vi "Set Legend (XYGraph).vi"(8 "error in (no error)":errorcluster, 9 "Plot.Plot Name":string, 10 "Active Plot":i32, 11 "XYGraph in":refnum<vi>) -> (0 "error out":errorcluster, 1 "Plot.Plot Name":string, 2 "Active Plot":i32, 3 "XYGraph out":refnum<vi>)   [LabVIEW 2019, in "Instrument UI.Lockin.lvclass"]
uses:
  Instrument UI.Lockin.lvclass
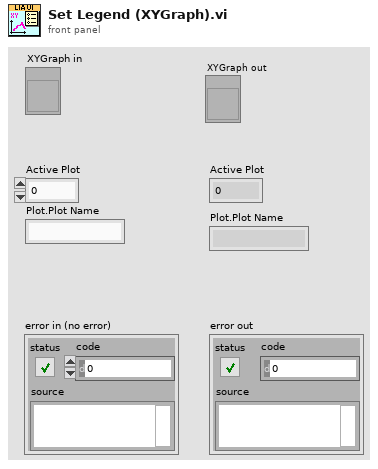
[diagram p1: front panel]
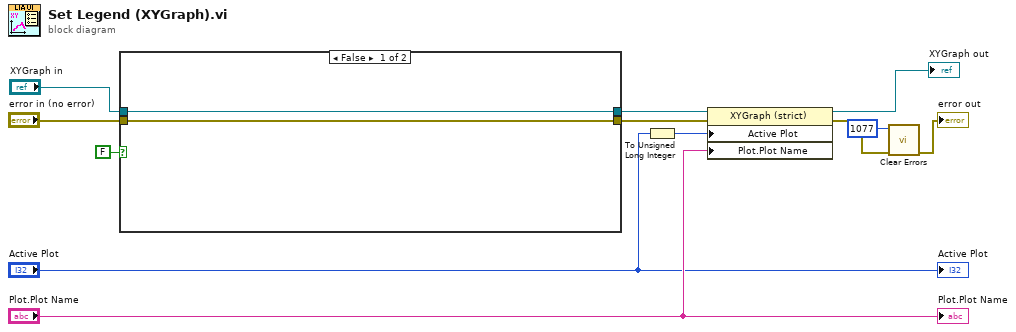
[diagram p0: block diagram]
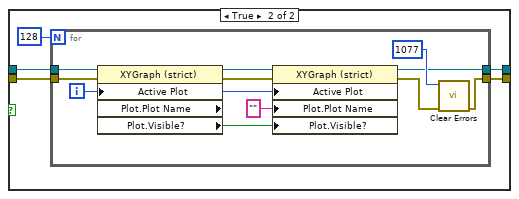
[diagram p2: hidden frame]
diagram:
  n1 = case shown="False" FALSE {
    tunnel: "XYGraph in" -> [w13 w16]
    tunnel: [w14 w19] -> w4
    tunnel: "error in (no error)" -> [w14 w18]
    tunnel: [w13 w15] -> w5
    frame False {
    }
    frame True {
      n2 = for {
        N: 128 -> [_]
        tunnel: w16 -> [w23]
        tunnel: [w28] -> w19
        tunnel: w18 -> [w22]
        tunnel: [w26] -> w15
        i -> [w21]
        n3 = property on="Property Node" class="XYGraph (strict)" props=["Active Plot", "Plot", "Plot Name", "Plot", "Visible?"](reference=w23, error in=w22, "Active Plot"=w21) -> (reference out=w25:refnum<vi>, error out=w24:errorcluster, "Plot.Visible?"=w20:bool)  [unwired: 1 out]
        n4 = property on="Property Node" class="XYGraph (strict)"(reference=w25, error in=w24, "Active Plot"=w21, "Plot.Plot Name"="" ("format string"), "Plot.Visible?"=w20) -> (reference out=w26:refnum<vi>, error out=w29:errorcluster)
        n5 = call <vilib>:"Clear Errors.vi"("error in (no error)"=w29, "specific error code to clear (0: all)"=1077) -> ("error out"=w28:errorcluster)  [unwired: 4 in, 1 out]
      }
    }
  }
  n6 = To Unsigned Long Integer(number="Active Plot") -> (unsigned 32bit integer=w3:u32)
  n7 = property on="Property Node" class="XYGraph (strict)"(reference=w5, error in=w4, "Active Plot"=w3, "Plot.Plot Name"="Plot.Plot Name") -> (reference out=→"XYGraph out":refnum<vi>, error out=w11:errorcluster)
  n8 = call <vilib>:"Clear Errors.vi"("error in (no error)"=w11, "specific error code to clear (0: all)"=1077) -> ("error out"=→"error out":errorcluster)  [unwired: 4 in, 1 out]
  "Active Plot" <- "Active Plot"
  "Plot.Plot Name" <- "Plot.Plot Name"
